vi "Update DatabaseP.vi"(9 "Amplitudes":string[](array[string]), 10 "Frequencies":string[](array[string]), 11 "DC_SN":string) -> ()   [LabVIEW 2024]
panel:
  out "Time Measured":string
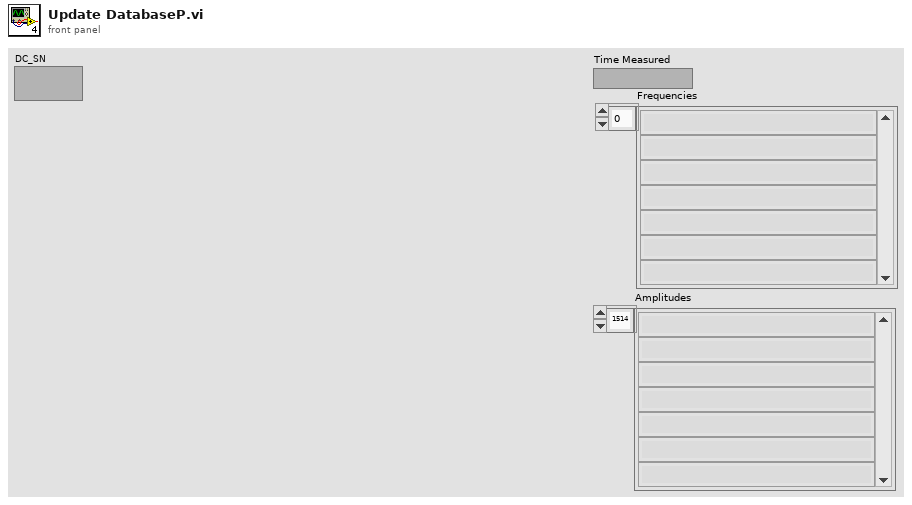
[diagram p1: front panel]
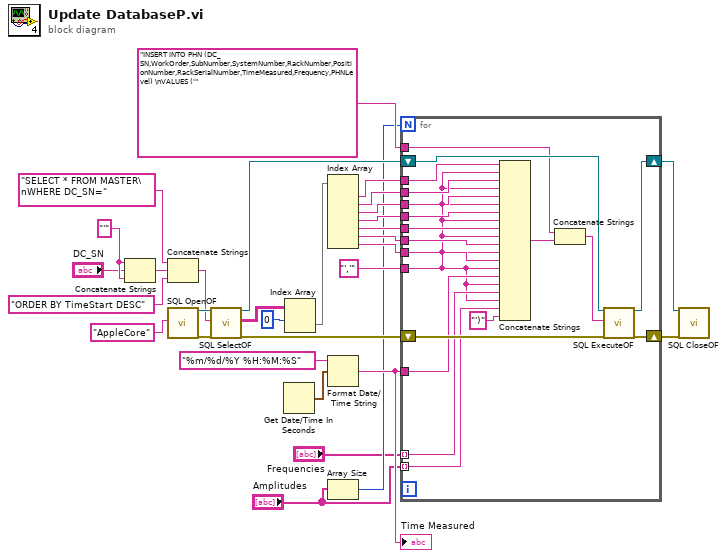
[diagram p0: block diagram]
diagram:
  w6 = "'" ("string")
  n1 = Concatenate Strings(w6, "DC_SN", w6) -> (w5:string)
  n2 = Concatenate Strings("SELECT * FROM MASTER\nWHERE DC_SN=" ("SQL Query"), w5, "ORDER BY TimeStart DESC" ("string")) -> (w17:string)
  n3 = call "SQL OpenOF.vi"("ConnectionString In"="AppleCore") -> ("Connection Out"=w30:refnum<k7>, "Error out"=w31:errorcluster)  [unwired: 17 in]
  n4 = call "SQL SelectOF.vi"("Connection In"=w30, "SQL Query"=w17, "Error in (no error)"=w31) -> ("Connection Out"=w28:refnum<k7>, "Data"=w18:string[][], "Error out"=w27:errorcluster)  [unwired: 14 in]
  n5 = Get Date/Time In Seconds() -> (seconds since 1Jan1904=w22:timestamp)
  n6 = Index Array(array=w18, index (row)=0 ("disabled index (row)")) -> (element=w19:string[])  [unwired: 1 in]
  n7 = Index Array(array=w19) -> (element #1=w16:string, element #2=w15:string, element #3=w14:string, element #4=w13:string, element #5=w12:string, element #6=w11:string, element #7=w10:string)  [unwired: 7 in]
  n8 = Format Date/Time String(time format string (%c)="%m/%d/%Y %H:%M:%S", seconds (now)=w22) -> (date/time string=w9:string)  [unwired: 1 in]
  "Time Measured" <- w9
  n9 = Array Size(array="Amplitudes") -> (size(s)=w3:i32)
  n10 = for {
    N: w3 -> [_]
    tunnel: w16 -> [w46]
    tunnel: w15 -> [w45]
    tunnel: w14 -> [w44]
    tunnel: w13 -> [w43]
    tunnel: w12 -> [w42]
    tunnel: w11 -> [w41]
    tunnel: w10 -> [w40]
    tunnel: w9 -> [w39]
    tunnel: "INSERT INTO PHN (DC_SN,WorkOrder,SubNumber,SystemNumber,RackNumber,PositionNumber,RackSerialNumber,TimeMeasured,Frequency,PHNLevel) \nVALUES ('" ("string") -> [w37]
    tunnel: "','" -> [w32]
    shift-right: [w48] -> w26
    shift-left: w28 -> [w50]
    shift-right: [w47] -> w25
    shift-left: w27 -> [w49]
    tunnel: "Frequencies" -> [w35] mode=indexing
    tunnel: "Amplitudes" -> [w34] mode=indexing
    n11 = Concatenate Strings(w46, w32, w45, w32, w44, w32, w43, w32, w42, w32, w41, w32, w40, w32, w39, w32, w35, w32, w34, "')" ("string")) -> (w38:string)
    n12 = Concatenate Strings(w37, w38) -> (w36:string)
    n13 = call "SQL ExecuteOF.vi"("Connection In"=w50, "SQL Query"=w36, "Error in (no error)"=w49) -> ("Connection Out"=w48:refnum<k7>, "Error out"=w47:errorcluster)  [unwired: 15 in]
  }
  n14 = call "SQL CloseOF.vi"("Connection In"=w26, "Error in (no error)"=w25) -> ()  [unwired: 17 in, 1 out]
